vi "ScheduledExitMessage_Send.vi"(8 "error in (no error)":errorcluster, 10 "scheduled exit reason":string, 11 "Qbus in":refnum<class "Qbus.lvclass">) -> (0 "error out":errorcluster, 3 "Qbus out":refnum<class "Qbus.lvclass">)   [LabVIEW 2017, in "Controller.lvlib"]
uses:
  <vilib>/addons/InsightCM/Devices/Shared/Common/Controller/Controller.lvlib
  <vilib>/addons/Qbus/Qbus.lvclass
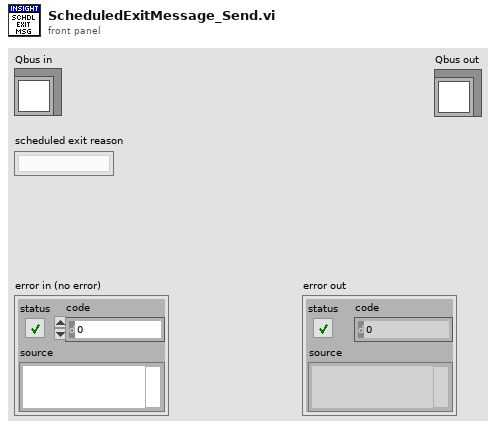
[diagram p1: front panel]
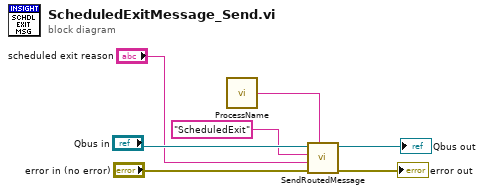
[diagram p0: block diagram]
diagram:
  n1 = call <vilib>:"ProcessName.vi"() -> ("ProcessName"=w3:string)  [unwired: 5 in]
  n2 = call <vilib>:"SendRoutedMessage.vi"("listener process"=w3, "error in (no error)"="error in (no error)", "message value"="scheduled exit reason", "message name"="ScheduledExit", "Qbus in"="Qbus in") -> ("error in (no error)"=→"error out":errorcluster, "Qbus out"=→"Qbus out":refnum<class "Qbus.lvclass">)  [unwired: 5 in]
